vi "Write unit ID.vi"(8 "error in (no error)":errorcluster caption="错误输入（无错误）", 10 "unit ID":u8, 11 "Standard Data Model in":refnum<class "Standard Data Model.lvclass">) -> (0 "error out":errorcluster caption="错误输出", 3 "Standard Data Model out":refnum<class "Standard Data Model.lvclass">)   [LabVIEW 2013, in "Modbus Library - Advance.lvlib" / "Standard Data Model.lvclass"]
uses:
  Standard Data Model.lvclass
  Standard Data Model.lvclass/Standard Data Model.ctl
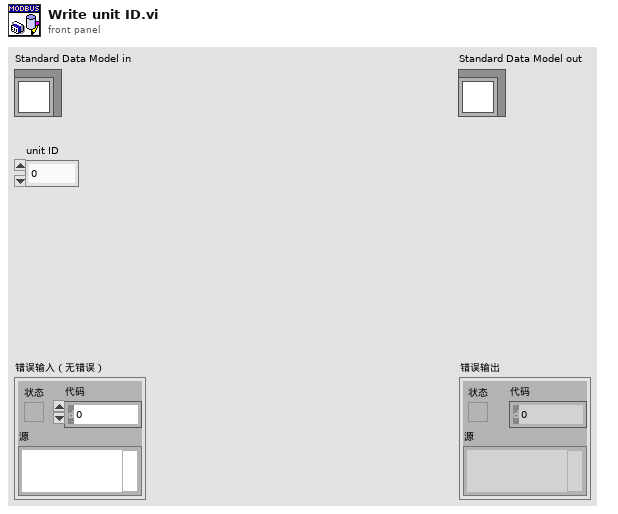
[diagram p1: front panel]
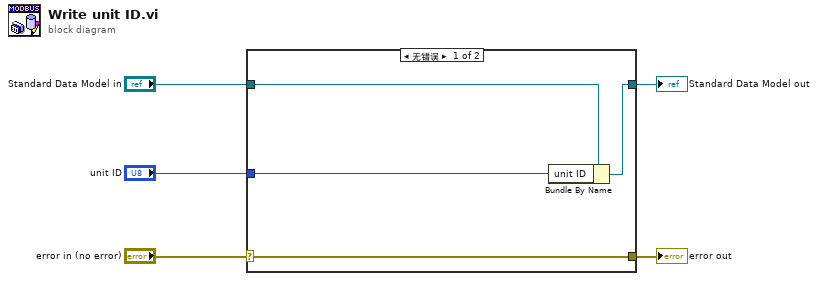
[diagram p0: block diagram]
diagram:
  n1 = case shown="无错误" "error in (no error)" {
    selector: "error in (no error)" -> [w9 w10]
    tunnel: [w9 w10] -> w4
    tunnel: [w7 w11] -> w2
    tunnel: "Standard Data Model in" -> [w8 w11]
    tunnel: "unit ID" -> [w6 _]
    frame No Error {
      n2 = Bundle By Name(cluster=w8, "unit ID"=w6) -> (w7:refnum<class "Standard Data Model.lvclass">)
    }
    frame Error {
    }
  }
  "error out" <- w4
  "Standard Data Model out" <- w2
